vi "SPAN Stufen abfragen Gasteiler.vi"(5 "GD Info Cluster":T1, 6 "Sprachliste":string[][](array[string]), 7 "Boolsche Stufen Flags Cluster":T11, 8 "error in (no error)":errorcluster caption="Fehler (Eingang, kein Fehler)", 9 "Index":T14, 10 "Referenzen Cluster":T12, 11 "SpanInletClusterArray in":T2[](array[typedef]) {"zusätzliche Zeitdauer Erster Punkt" min=30 step=1 format="%#_5g"; "Zeitdauer Stufen" format="%#_5g"; "Max Fehler" format="%#_5g"; "Anzahl Stufen" format="%#_5g"; "Komponenten"."Komponente 5"."Komponente:" items=["NO (350,3000) LP 191C", "NO2 (150) LP 191C (1of2)", "NO2 (2000) LP 191C (2of2)", "N2O (300) LP 191C (1of2)", "NH3 (300) LP 191C (1of2)", "NH3 (900,3000) LP 191C (2of2)", "HNCO (400) 191C", "H2O% (30) LP 191C", "Formaldehyde (70,500) LP 191C", "CO2 low% (4) LP 191C (2of2)", "CO2% (20) LP 191C (1of2)", "CO (700) LP 191C (1of3)", "CO% (1) LP 191C (2of3)", "Propylene (1000) LP 191C", "Aromatic HC C7 (500) LP 191C", "Ethylene (1000) LP 191C", "CH4 (250) LP 191C (1of2)", "CH4 (5000) LP 191C (2of2)", "Ethane (1000) LP 191C", "Acetylene (1000) LP 191C", "HNO2 (20) 191C", "MeOH (1000) 191C", "CO% (10) LP 191C (3of3)", "Formic Acid (100) 191C", "SO2 (500) LP 191C", "Acetaldehyde (1000) LP 191C", "COS (100) LP 191C", "1,3 butadiene (100) LP 191C", "Oil as Octane (200) LP 191C", "N2O (1000) LP 191C (2of2)", "Propane (200) LP 191C", "NO2 autorange (2000)", "CO autorange (100000)", "CH4 autorange (5000)", "NH3 autorange (3000)", "Temp. Gascell", "Pressure Gascell", "sBeam@2500"]; "Komponenten"."Komponente 5"."Konzentration IST" format="%#.4f"; "Komponenten"."Komponente 5"."Genauigkeit" format="%#.1f"; "Komponenten"."Komponente 4"."Komponente:" items=["NO (350,3000) LP 191C", "NO2 (150) LP 191C (1of2)", "NO2 (2000) LP 191C (2of2)", "N2O (300) LP 191C (1of2)", "NH3 (300) LP 191C (1of2)", "NH3 (900,3000) LP 191C (2of2)", "HNCO (400) 191C", "H2O% (30) LP 191C", "Formaldehyde (70,500) LP 191C", "CO2 low% (4) LP 191C (2of2)", "CO2% (20) LP 191C (1of2)", "CO (700) LP 191C (1of3)", "CO% (1) LP 191C (2of3)", "Propylene (1000) LP 191C", "Aromatic HC C7 (500) LP 191C", "Ethylene (1000) LP 191C", "CH4 (250) LP 191C (1of2)", "CH4 (5000) LP 191C (2of2)", "Ethane (1000) LP 191C", "Acetylene (1000) LP 191C", "HNO2 (20) 191C", "MeOH (1000) 191C", "CO% (10) LP 191C (3of3)", "Formic Acid (100) 191C", "SO2 (500) LP 191C", "Acetaldehyde (1000) LP 191C", "COS (100) LP 191C", "1,3 butadiene (100) LP 191C", "Oil as Octane (200) LP 191C", "N2O (1000) LP 191C (2of2)", "Propane (200) LP 191C", "NO2 autorange (2000)", "CO autorange (100000)", "CH4 autorange (5000)", "NH3 autorange (3000)", "Temp. Gascell", "Pressure Gascell", "sBeam@2500"]; "Komponenten"."Komponente 4"."Konzentration IST" format="%#.4f"; "Komponenten"."Komponente 4"."Genauigkeit" format="%#.1f"; "Komponenten"."Komponente 3"."Komponente:" items=["NO (350,3000) LP 191C", "NO2 (150) LP 191C (1of2)", "NO2 (2000) LP 191C (2of2)", "N2O (300) LP 191C (1of2)", "NH3 (300) LP 191C (1of2)", "NH3 (900,3000) LP 191C (2of2)", "HNCO (400) 191C", "H2O% (30) LP 191C", "Formaldehyde (70,500) LP 191C", "CO2 low% (4) LP 191C (2of2)", "CO2% (20) LP 191C (1of2)", "CO (700) LP 191C (1of3)", "CO% (1) LP 191C (2of3)", "Propylene (1000) LP 191C", "Aromatic HC C7 (500) LP 191C", "Ethylene (1000) LP 191C", "CH4 (250) LP 191C (1of2)", "CH4 (5000) LP 191C (2of2)", "Ethane (1000) LP 191C", "Acetylene (1000) LP 191C", "HNO2 (20) 191C", "MeOH (1000) 191C", "CO% (10) LP 191C (3of3)", "Formic Acid (100) 191C", "SO2 (500) LP 191C", "Acetaldehyde (1000) LP 191C", "COS (100) LP 191C", "1,3 butadiene (100) LP 191C", "Oil as Octane (200) LP 191C", "N2O (1000) LP 191C (2of2)", "Propane (200) LP 191C", "NO2 autorange (2000)", "CO autorange (100000)", "CH4 autorange (5000)", "NH3 autorange (3000)", "Temp. Gascell", "Pressure Gascell", "sBeam@2500"]; "Komponenten"."Komponente 3"."Konzentration IST" format="%#.4f"; "Komponenten"."Komponente 3"."Genauigkeit" format="%#.1f"; "Komponenten"."Komponente 2"."Komponente:" items=["NO (350,3000) LP 191C", "NO2 (150) LP 191C (1of2)", "NO2 (2000) LP 191C (2of2)", "N2O (300) LP 191C (1of2)", "NH3 (300) LP 191C (1of2)", "NH3 (900,3000) LP 191C (2of2)", "HNCO (400) 191C", "H2O% (30) LP 191C", "Formaldehyde (70,500) LP 191C", "CO2 low% (4) LP 191C (2of2)", "CO2% (20) LP 191C (1of2)", "CO (700) LP 191C (1of3)", "CO% (1) LP 191C (2of3)", "Propylene (1000) LP 191C", "Aromatic HC C7 (500) LP 191C", "Ethylene (1000) LP 191C", "CH4 (250) LP 191C (1of2)", "CH4 (5000) LP 191C (2of2)", "Ethane (1000) LP 191C", "Acetylene (1000) LP 191C", "HNO2 (20) 191C", "MeOH (1000) 191C", "CO% (10) LP 191C (3of3)", "Formic Acid (100) 191C", "SO2 (500) LP 191C", "Acetaldehyde (1000) LP 191C", "COS (100) LP 191C", "1,3 butadiene (100) LP 191C", "Oil as Octane (200) LP 191C", "N2O (1000) LP 191C (2of2)", "Propane (200) LP 191C", "NO2 autorange (2000)", "CO autorange (100000)", "CH4 autorange (5000)", "NH3 autorange (3000)", "Temp. Gascell", "Pressure Gascell", "sBeam@2500"]; "Komponenten"."Komponente 2"."Konzentration IST" format="%#.4f"; "Komponenten"."Komponente 2"."Genauigkeit" format="%#.1f"; "Komponenten"."Komponente 1"."Komponente:" items=["NO (350,3000) LP 191C", "NO2 (150) LP 191C (1of2)", "NO2 (2000) LP 191C (2of2)", "N2O (300) LP 191C (1of2)", "NH3 (300) LP 191C (1of2)", "NH3 (900,3000) LP 191C (2of2)", "HNCO (400) 191C", "H2O% (30) LP 191C", "Formaldehyde (70,500) LP 191C", "CO2 low% (4) LP 191C (2of2)", "CO2% (20) LP 191C (1of2)", "CO (700) LP 191C (1of3)", "CO% (1) LP 191C (2of3)", "Propylene (1000) LP 191C", "Aromatic HC C7 (500) LP 191C", "Ethylene (1000) LP 191C", "CH4 (250) LP 191C (1of2)", "CH4 (5000) LP 191C (2of2)", "Ethane (1000) LP 191C", "Acetylene (1000) LP 191C", "HNO2 (20) 191C", "MeOH (1000) 191C", "CO% (10) LP 191C (3of3)", "Formic Acid (100) 191C", "SO2 (500) LP 191C", "Acetaldehyde (1000) LP 191C", "COS (100) LP 191C", "1,3 butadiene (100) LP 191C", "Oil as Octane (200) LP 191C", "N2O (1000) LP 191C (2of2)", "Propane (200) LP 191C", "NO2 autorange (2000)", "CO autorange (100000)", "CH4 autorange (5000)", "NH3 autorange (3000)", "Temp. Gascell", "Pressure Gascell", "sBeam@2500"]; "Komponenten"."Komponente 1"."Konzentration IST" format="%#.4f"; "Komponenten"."Komponente 1"."Genauigkeit" format="%#.1f"; "Ablaufdatum" format="%<%d.%m.%Y>T"; "Gasflasche" items=["----"=10000, "IAG NH3 3000"=0, "IAG NH3 200"=1, "IAG NH3 2000"=2, "IAG MG"=3, "IAG O2"=4]}) -> (0 "error out":errorcluster caption="Fehler (Ausgang)", 1 "Component Index out":i32, 2 "SPAN Index out":i32, 3 "SpanInletClusterArray out":T2[](array[typedef]) {"zusätzliche Zeitdauer Erster Punkt" min=30 step=1 format="%#_5g"; "Zeitdauer Stufen" format="%#_5g"; "Max Fehler" format="%#_5g"; "Anzahl Stufen" format="%#_5g"; "Komponenten"."Komponente 5"."Komponente:" items=["NO (350,3000) LP 191C", "NO2 (150) LP 191C (1of2)", "NO2 (2000) LP 191C (2of2)", "N2O (300) LP 191C (1of2)", "NH3 (300) LP 191C (1of2)", "NH3 (900,3000) LP 191C (2of2)", "HNCO (400) 191C", "H2O% (30) LP 191C", "Formaldehyde (70,500) LP 191C", "CO2 low% (4) LP 191C (2of2)", "CO2% (20) LP 191C (1of2)", "CO (700) LP 191C (1of3)", "CO% (1) LP 191C (2of3)", "Propylene (1000) LP 191C", "Aromatic HC C7 (500) LP 191C", "Ethylene (1000) LP 191C", "CH4 (250) LP 191C (1of2)", "CH4 (5000) LP 191C (2of2)", "Ethane (1000) LP 191C", "Acetylene (1000) LP 191C", "HNO2 (20) 191C", "MeOH (1000) 191C", "CO% (10) LP 191C (3of3)", "Formic Acid (100) 191C", "SO2 (500) LP 191C", "Acetaldehyde (1000) LP 191C", "COS (100) LP 191C", "1,3 butadiene (100) LP 191C", "Oil as Octane (200) LP 191C", "N2O (1000) LP 191C (2of2)", "Propane (200) LP 191C", "NO2 autorange (2000)", "CO autorange (100000)", "CH4 autorange (5000)", "NH3 autorange (3000)", "Temp. Gascell", "Pressure Gascell", "sBeam@2500"]; "Komponenten"."Komponente 5"."Konzentration IST" format="%#.4f"; "Komponenten"."Komponente 5"."Genauigkeit" format="%#.1f"; "Komponenten"."Komponente 4"."Komponente:" items=["NO (350,3000) LP 191C", "NO2 (150) LP 191C (1of2)", "NO2 (2000) LP 191C (2of2)", "N2O (300) LP 191C (1of2)", "NH3 (300) LP 191C (1of2)", "NH3 (900,3000) LP 191C (2of2)", "HNCO (400) 191C", "H2O% (30) LP 191C", "Formaldehyde (70,500) LP 191C", "CO2 low% (4) LP 191C (2of2)", "CO2% (20) LP 191C (1of2)", "CO (700) LP 191C (1of3)", "CO% (1) LP 191C (2of3)", "Propylene (1000) LP 191C", "Aromatic HC C7 (500) LP 191C", "Ethylene (1000) LP 191C", "CH4 (250) LP 191C (1of2)", "CH4 (5000) LP 191C (2of2)", "Ethane (1000) LP 191C", "Acetylene (1000) LP 191C", "HNO2 (20) 191C", "MeOH (1000) 191C", "CO% (10) LP 191C (3of3)", "Formic Acid (100) 191C", "SO2 (500) LP 191C", "Acetaldehyde (1000) LP 191C", "COS (100) LP 191C", "1,3 butadiene (100) LP 191C", "Oil as Octane (200) LP 191C", "N2O (1000) LP 191C (2of2)", "Propane (200) LP 191C", "NO2 autorange (2000)", "CO autorange (100000)", "CH4 autorange (5000)", "NH3 autorange (3000)", "Temp. Gascell", "Pressure Gascell", "sBeam@2500"]; "Komponenten"."Komponente 4"."Konzentration IST" format="%#.4f"; "Komponenten"."Komponente 4"."Genauigkeit" format="%#.1f"; "Komponenten"."Komponente 3"."Komponente:" items=["NO (350,3000) LP 191C", "NO2 (150) LP 191C (1of2)", "NO2 (2000) LP 191C (2of2)", "N2O (300) LP 191C (1of2)", "NH3 (300) LP 191C (1of2)", "NH3 (900,3000) LP 191C (2of2)", "HNCO (400) 191C", "H2O% (30) LP 191C", "Formaldehyde (70,500) LP 191C", "CO2 low% (4) LP 191C (2of2)", "CO2% (20) LP 191C (1of2)", "CO (700) LP 191C (1of3)", "CO% (1) LP 191C (2of3)", "Propylene (1000) LP 191C", "Aromatic HC C7 (500) LP 191C", "Ethylene (1000) LP 191C", "CH4 (250) LP 191C (1of2)", "CH4 (5000) LP 191C (2of2)", "Ethane (1000) LP 191C", "Acetylene (1000) LP 191C", "HNO2 (20) 191C", "MeOH (1000) 191C", "CO% (10) LP 191C (3of3)", "Formic Acid (100) 191C", "SO2 (500) LP 191C", "Acetaldehyde (1000) LP 191C", "COS (100) LP 191C", "1,3 butadiene (100) LP 191C", "Oil as Octane (200) LP 191C", "N2O (1000) LP 191C (2of2)", "Propane (200) LP 191C", "NO2 autorange (2000)", "CO autorange (100000)", "CH4 autorange (5000)", "NH3 autorange (3000)", "Temp. Gascell", "Pressure Gascell", "sBeam@2500"]; "Komponenten"."Komponente 3"."Konzentration IST" format="%#.4f"; "Komponenten"."Komponente 3"."Genauigkeit" format="%#.1f"; "Komponenten"."Komponente 2"."Komponente:" items=["NO (350,3000) LP 191C", "NO2 (150) LP 191C (1of2)", "NO2 (2000) LP 191C (2of2)", "N2O (300) LP 191C (1of2)", "NH3 (300) LP 191C (1of2)", "NH3 (900,3000) LP 191C (2of2)", "HNCO (400) 191C", "H2O% (30) LP 191C", "Formaldehyde (70,500) LP 191C", "CO2 low% (4) LP 191C (2of2)", "CO2% (20) LP 191C (1of2)", "CO (700) LP 191C (1of3)", "CO% (1) LP 191C (2of3)", "Propylene (1000) LP 191C", "Aromatic HC C7 (500) LP 191C", "Ethylene (1000) LP 191C", "CH4 (250) LP 191C (1of2)", "CH4 (5000) LP 191C (2of2)", "Ethane (1000) LP 191C", "Acetylene (1000) LP 191C", "HNO2 (20) 191C", "MeOH (1000) 191C", "CO% (10) LP 191C (3of3)", "Formic Acid (100) 191C", "SO2 (500) LP 191C", "Acetaldehyde (1000) LP 191C", "COS (100) LP 191C", "1,3 butadiene (100) LP 191C", "Oil as Octane (200) LP 191C", "N2O (1000) LP 191C (2of2)", "Propane (200) LP 191C", "NO2 autorange (2000)", "CO autorange (100000)", "CH4 autorange (5000)", "NH3 autorange (3000)", "Temp. Gascell", "Pressure Gascell", "sBeam@2500"]; "Komponenten"."Komponente 2"."Konzentration IST" format="%#.4f"; "Komponenten"."Komponente 2"."Genauigkeit" format="%#.1f"; "Komponenten"."Komponente 1"."Komponente:" items=["NO (350,3000) LP 191C", "NO2 (150) LP 191C (1of2)", "NO2 (2000) LP 191C (2of2)", "N2O (300) LP 191C (1of2)", "NH3 (300) LP 191C (1of2)", "NH3 (900,3000) LP 191C (2of2)", "HNCO (400) 191C", "H2O% (30) LP 191C", "Formaldehyde (70,500) LP 191C", "CO2 low% (4) LP 191C (2of2)", "CO2% (20) LP 191C (1of2)", "CO (700) LP 191C (1of3)", "CO% (1) LP 191C (2of3)", "Propylene (1000) LP 191C", "Aromatic HC C7 (500) LP 191C", "Ethylene (1000) LP 191C", "CH4 (250) LP 191C (1of2)", "CH4 (5000) LP 191C (2of2)", "Ethane (1000) LP 191C", "Acetylene (1000) LP 191C", "HNO2 (20) 191C", "MeOH (1000) 191C", "CO% (10) LP 191C (3of3)", "Formic Acid (100) 191C", "SO2 (500) LP 191C", "Acetaldehyde (1000) LP 191C", "COS (100) LP 191C", "1,3 butadiene (100) LP 191C", "Oil as Octane (200) LP 191C", "N2O (1000) LP 191C (2of2)", "Propane (200) LP 191C", "NO2 autorange (2000)", "CO autorange (100000)", "CH4 autorange (5000)", "NH3 autorange (3000)", "Temp. Gascell", "Pressure Gascell", "sBeam@2500"]; "Komponenten"."Komponente 1"."Konzentration IST" format="%#.4f"; "Komponenten"."Komponente 1"."Genauigkeit" format="%#.1f"; "Ablaufdatum" format="%<%d.%m.%Y>T"; "Gasflasche" items=["----"=10000, "IAG NH3 3000"=0, "IAG NH3 200"=1, "IAG NH3 2000"=2, "IAG MG"=3, "IAG O2"=4]}, 4 "Status out":string)   [LabVIEW 2020, in "Linearisierung v2.lvlib" / "SpanEinstellungen.lvlib"]
uses:
  SpanEinstellungen.lvlib
  Visualisierungs Elemente/Checkbox(boolsch).ctl
  GD Abfrage Referenzen.ctl
  Boolsche Stufen Flags.ctl
  SpanInletCluster.ctl
  Seiten/System Einstellungen V2/Konfig Gasflasche.ctl
  Seiten/System Einstellungen V2/Analysatoren.ctl
  Seiten/System Einstellungen V2/Gasflasche Auswahl.ctl
  Komponentencluster mit Formel.ctl
  Komponentenauswahl mit Formel.ctl
  Visualisierungs Elemente/String - Eingabefeld.ctl
  Einheit.ctl
  Seiten/System Einstellungen V2/Traegergas.ctl
  GasteilerType.ctl
  Gasteiler/Aktionen FGV Gasteiler Daten.ctl
  Linearisierung v2.lvlib
  Gasteiler/Gasteiler.lvlib
  Sprachverwaltung/Sprachverwaltung.lvlib
  Seiten/System Einstellungen V2/System Einstellungen V2.lvlib
panel:
  # "sec"
  # "%"
  # "sec"
  # "Komponente"
  # "Formel"
  # "Konzentration"
  # "Einheit"
  # "Genauigkeit [%]"
  # "sec"
  # "%"
  # "sec"
  # "Komponente"
  # "Formel"
  # "Konzentration"
  # "Einheit"
  # "Genauigkeit [%]"
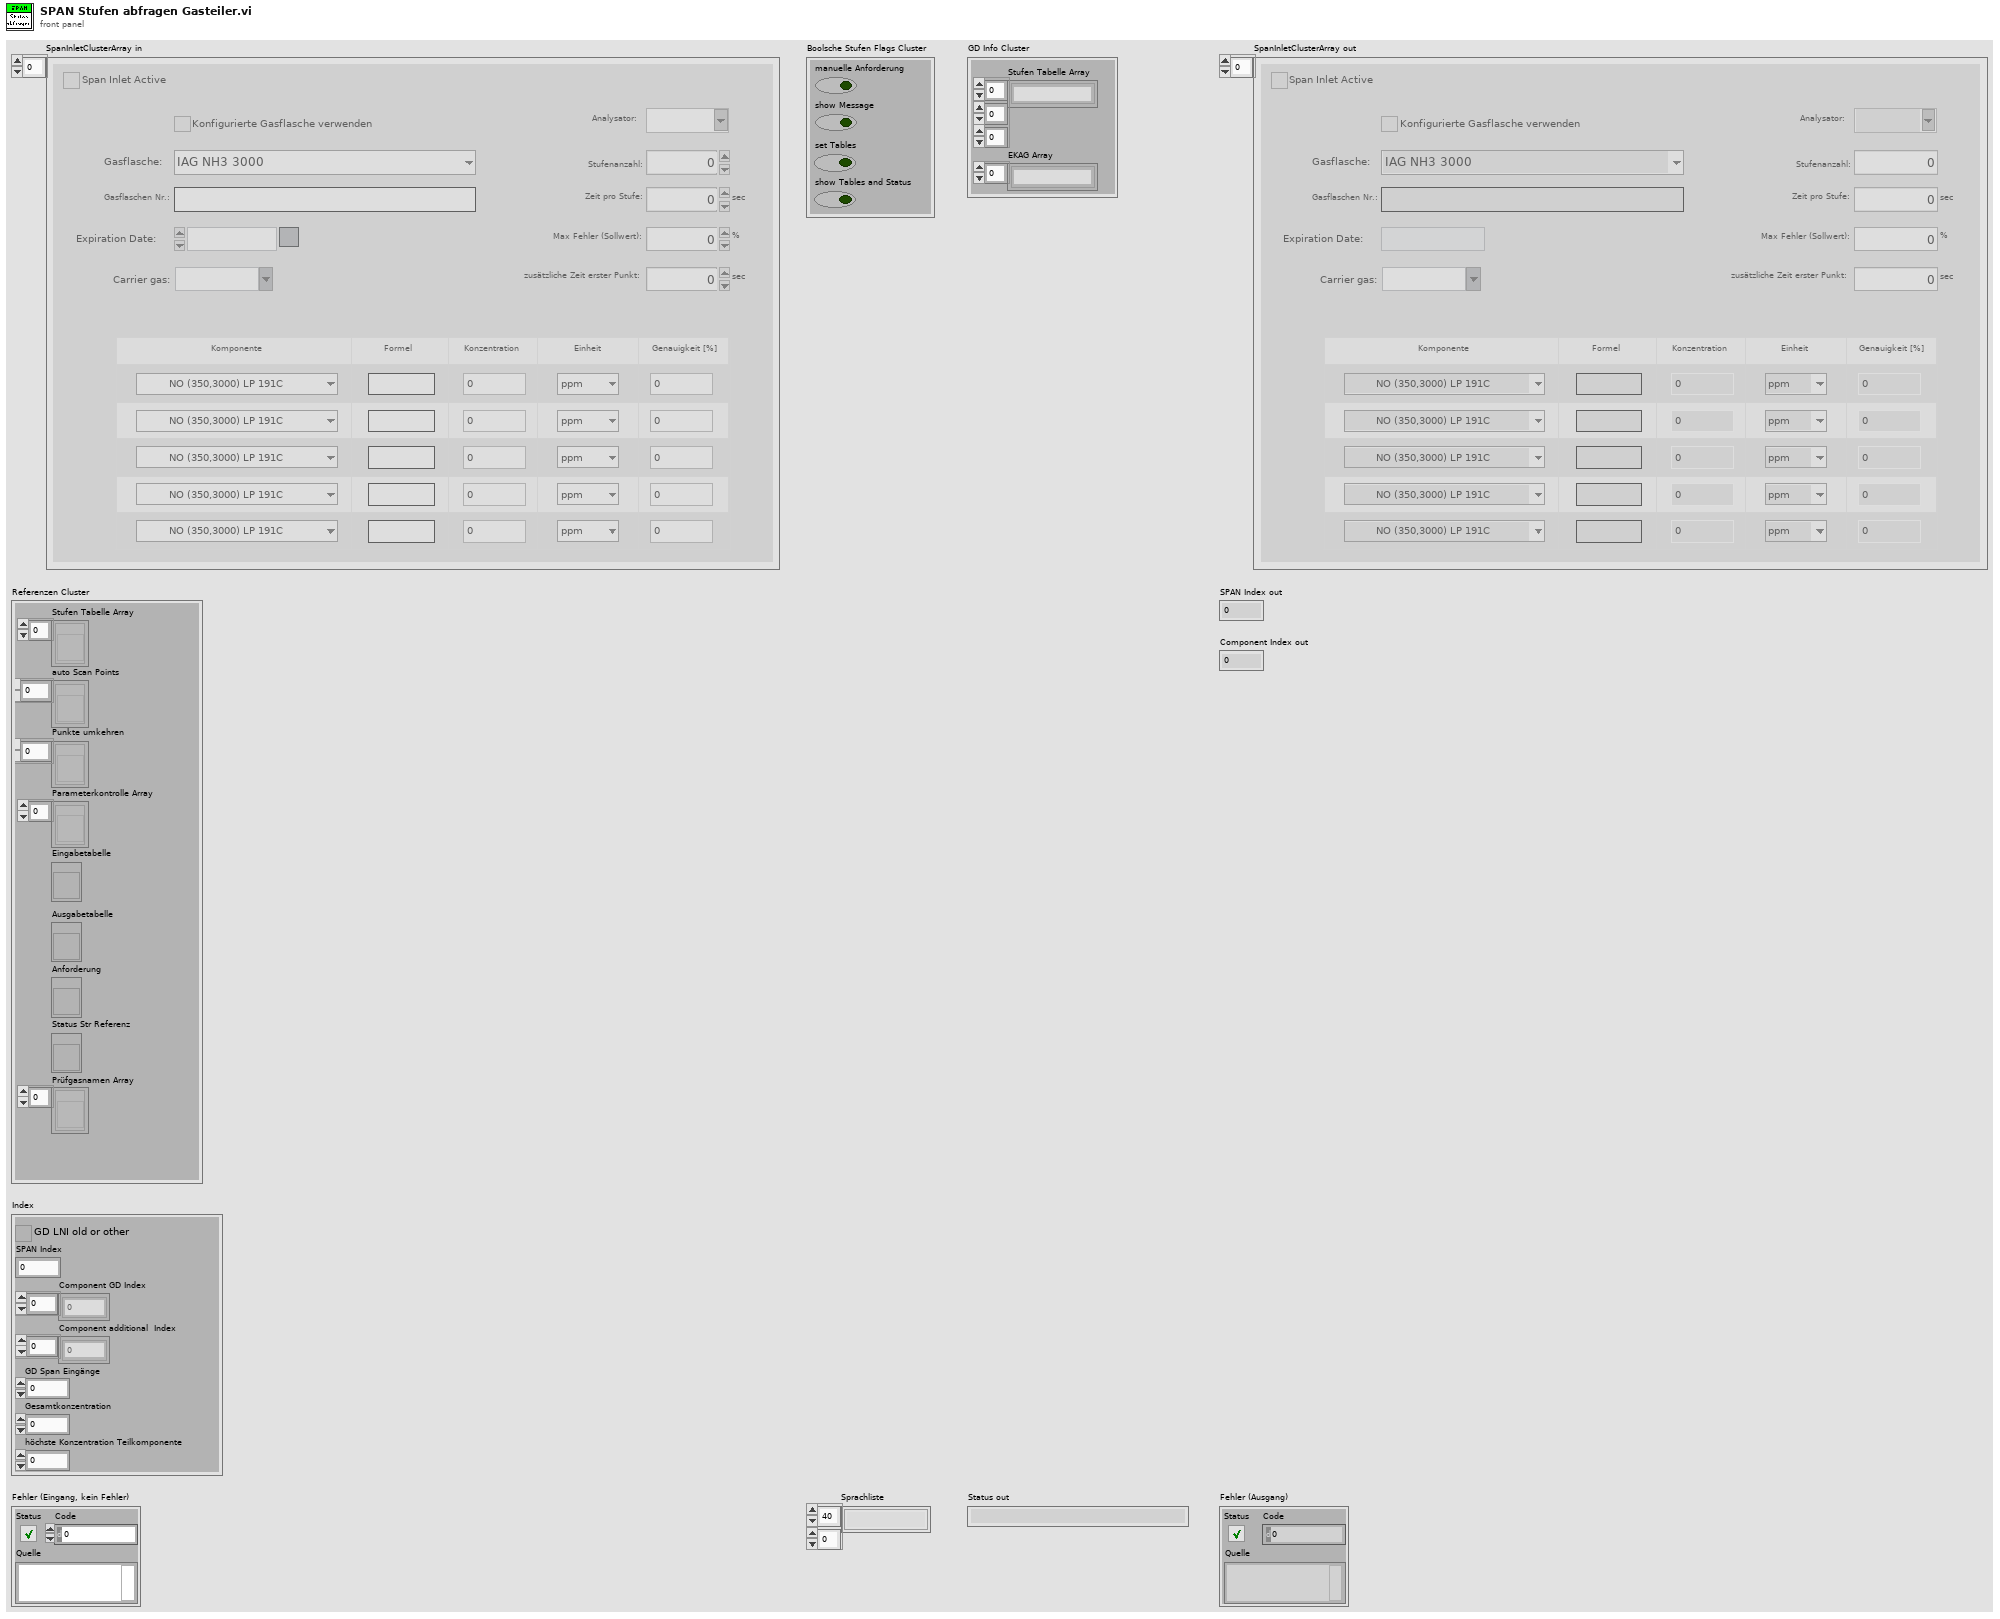
[diagram p1: front panel]
types:
  T1 = cluster{"Stufen Tabelle Array":string[][][], "EKAG Array":string[]}
  T2 = typedef "Linearisierung v2.lvlib/SpanEinstellungen.lvlib/SpanInletCluster.ctl" = cluster{"Span Inlet Active":T3, "Analysator":T4, "Konfig Gasflasche":T3, "Gasflasche":T5, "Gasflaschen Nr.:":string, "Ablaufdatum":timestamp, "Komponenten":T6, "Zeitdauer Stufen":sgl, "Max Fehler":sgl, "Anzahl Stufen":sgl, "Trägergas":T10, "zusätzliche Zeitdauer Erster Punkt":sgl}
  T3 = typedef "System Einstellungen V2.lvlib/Konfig Gasflasche.ctl" = bool
  T4 = typedef "System Einstellungen V2.lvlib/Analysatoren.ctl" = string
  T5 = typedef "System Einstellungen V2.lvlib/Gasflasche Auswahl.ctl" = u16
  T6 = typedef "Linearisierung v2.lvlib/SpanEinstellungen.lvlib/Komponentencluster mit Formel.ctl" = cluster{"Komponente 1":T7, "Komponente 2":T7, "Komponente 3":T7, "Komponente 4":T7, "Komponente 5":T7}
  T7 = typedef "Linearisierung v2.lvlib/SpanEinstellungen.lvlib/Komponentenauswahl mit Formel.ctl" = cluster{"Komponente:":u16, "Summenformel":T8, "Konzentration IST":dbl, "Einheit":T9, "Genauigkeit":dbl}
  T8 = typedef "String - Eingabefeld.ctl" = string
  T9 = typedef "Linearisierung v2.lvlib/SpanEinstellungen.lvlib/Einheit.ctl" = enum16{"ppm", "%"}
  T10 = typedef "System Einstellungen V2.lvlib/Traegergas.ctl" = string
  T11 = typedef "Linearisierung v2.lvlib/SpanEinstellungen.lvlib/Boolsche Stufen Flags.ctl" = cluster{"manuelle Anforderung":bool, "show Message":bool, "set Tables":bool, "show Tables and Status":bool}
  T12 = typedef "Linearisierung v2.lvlib/SpanEinstellungen.lvlib/GD Abfrage Referenzen.ctl" = cluster{"Stufen Tabelle Array":refnum<vi>[], "auto Scan Points":refnum<vi>[], "Punkte umkehren":refnum<vi>[], "Parameterkontrolle Array":refnum<vi>[], "Eingabetabelle":refnum<vi>, "Ausgabetabelle":refnum<vi>, "Anforderung":refnum<vi>, "Status Str Referenz":refnum<vi>, "Prüfgasnamen Array":refnum<vi>[]}
  T13 = typedef "Checkbox(boolsch).ctl" = bool
  T14 = cluster{"GD LNI old or other":T13, "SPAN Index":i32, "Component GD Index":i32[], "Component additional  Index":i32[], "GD Span Eingänge":u16, "Gesamtkonzentration":dbl, "höchste Konzentration Teilkomponente":dbl}
  T15 = typedef "Linearisierung v2.lvlib/Gasteiler.lvlib/Aktionen FGV Gasteiler Daten.ctl" = enum16{"lesen", "Gasteiler Daten", "Seriellen Param.", "MB-Endwert", "laden", "speichern", "Anforderung", "TCP", "Aufzeichnung Start"}
  T16 = typedef "Linearisierung v2.lvlib/GasteilerType.ctl" = u16
  T17 = typedef "Linearisierung v2.lvlib/Gasteiler.lvlib/Gasteiler Daten.ctl" = cluster{"Gasteiler":T8, "Gasteiler Stufen":T18, "Gasteiler Type":T16, "Konfig Gasteiler":T19, "Gasteiler Span Eingänge":u16}
  T18 = typedef "Linearisierung v2.lvlib/Gasteiler.lvlib/Gasteiler Stufen.ctl" = u16
  T19 = typedef "System Einstellungen V2.lvlib/Gasteiler Auswahl.ctl" = u16
  T20 = typedef "Button.ctl" = bool
  T21 = cluster{"Komponente:":u16, "Konzentration IST":dbl}[]
  T22 = typedef "Linearisierung v2.lvlib/Gasteiler.lvlib/Prüfgas in.ctl" = u16
  T23 = cluster{"GD LNI old or other":T13, "Anzahl Stufen":sgl, "Verdünnungsgas":T22, "Component GD Index":i32[], "Component additional  Index":i32[], "DIL Input":i32}
  T24 = cluster{"manuelle Anforderung":bool, "show Tables and Status":bool}
  T25 = cluster{"Stufen Tabellen out":string[][][], "EGAK":T10[], "AGAK":string[]}
  T26 = cluster{"SPAN Index":i32, "Component Index out":i32}
  T27 = cluster{i32, cluster{"SPAN Index":i32, "Component Index out":i32}}
  T28 = cluster{bool, bool, "Gesamtkonzentration":dbl, "höchste Konzentration Teilkomponente":dbl}
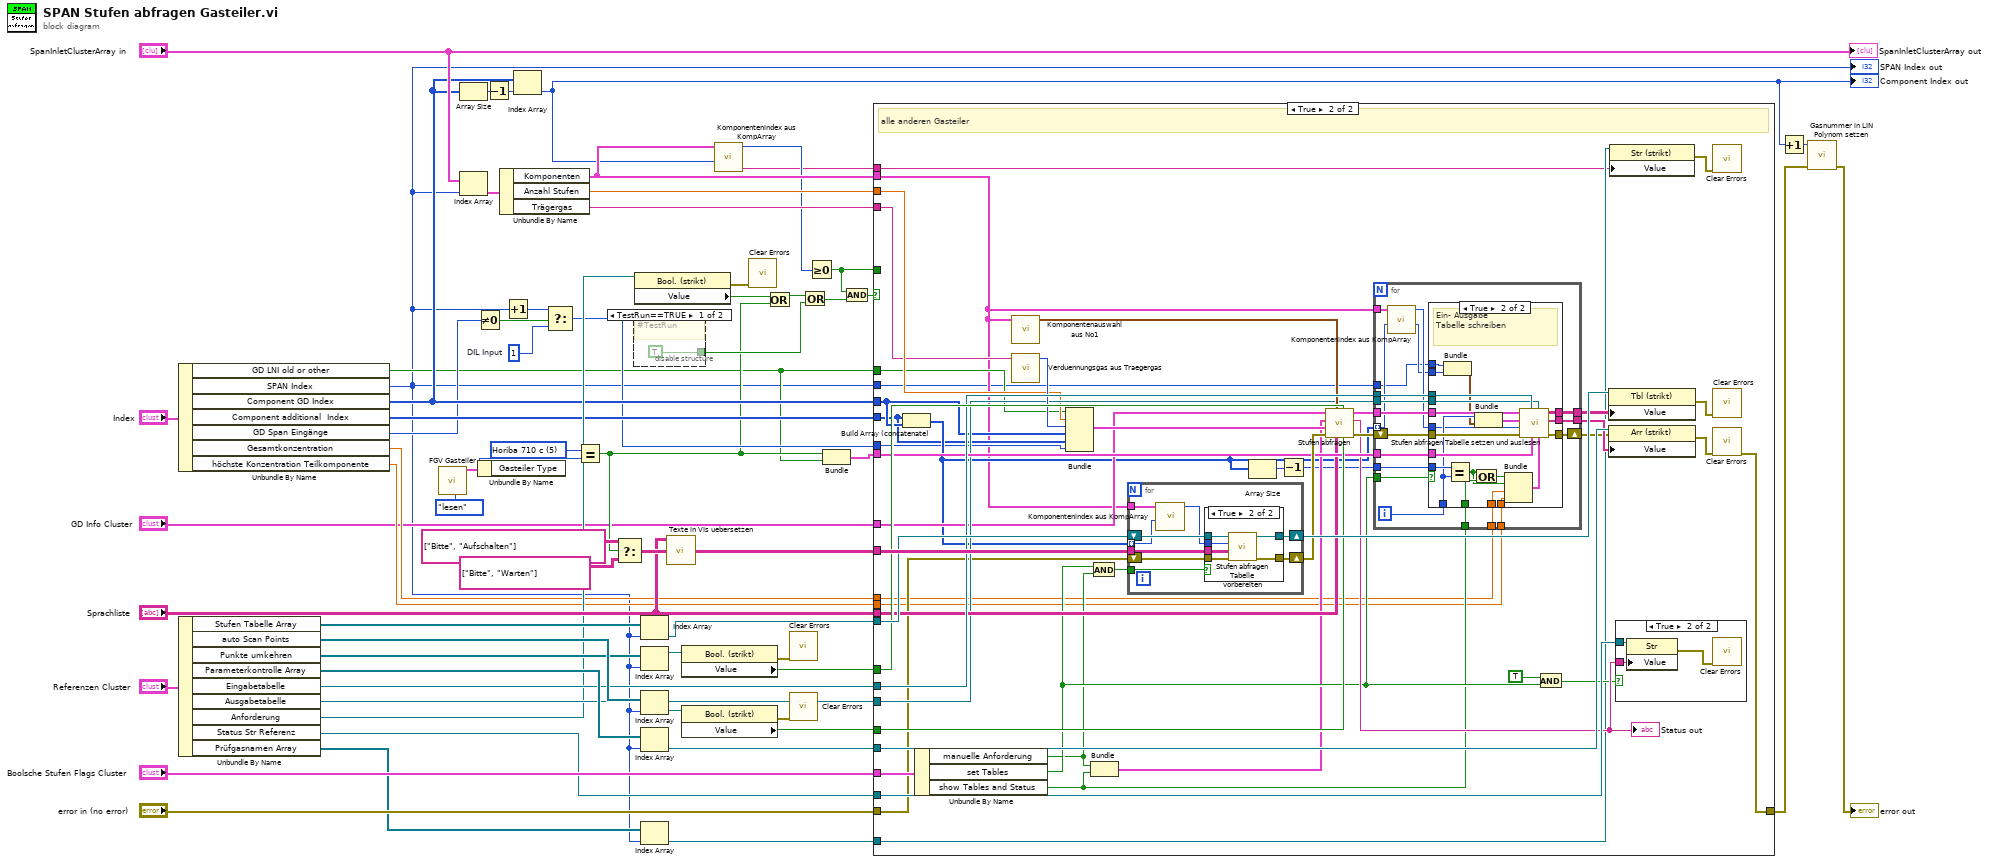
[diagram p0: block diagram]
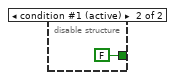
[diagram p2: hidden frame]
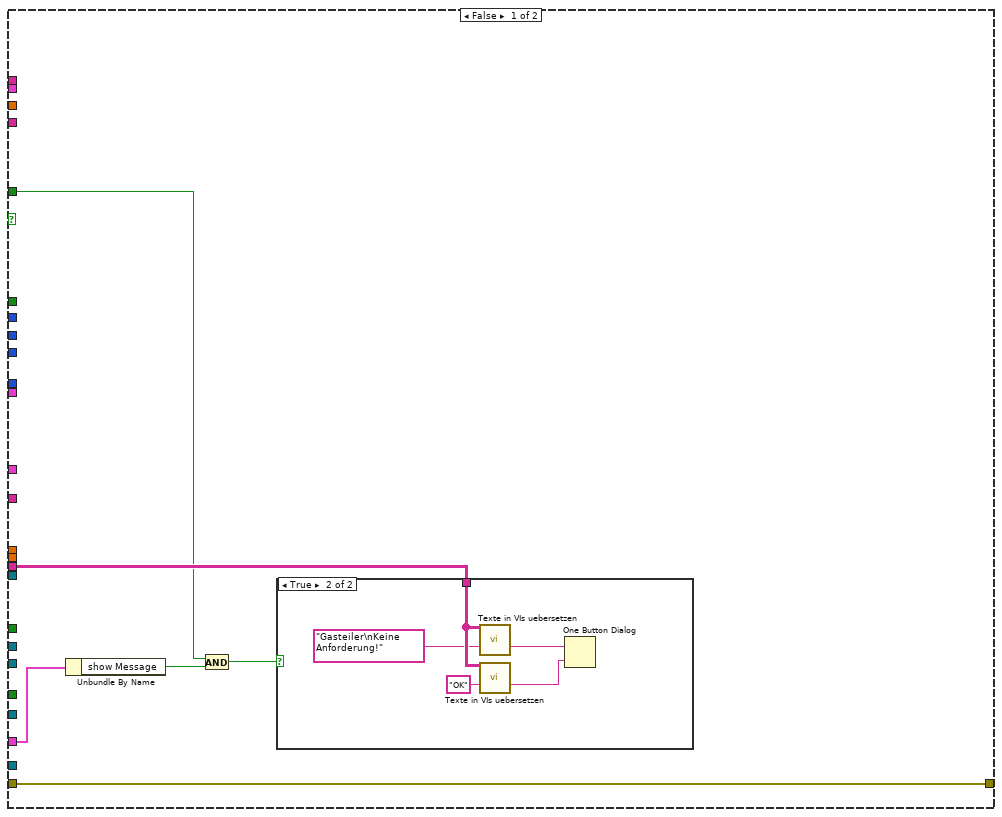
[diagram p3: hidden frame]
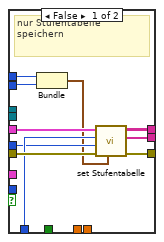
[diagram p5: hidden frame]
diagram:
  w17 = 1  # DIL Input
  w61 = T16 5 items=["LCD-Touch-Display", "Analog-Display", "AVL GDU", "Horiba GDC", "HovaCal", "Horiba 710 c"] ("x")
  n1 = Unbundle By Name("Index") -> ("GD LNI old or other"=w5:T13, "SPAN Index"=w1:i32, "Component GD Index"=w24:i32[], "Component additional  Index"=w25:i32[], "GD Span Eingänge"=w19:u16, "Gesamtkonzentration"=w12:dbl, "höchste Konzentration Teilkomponente"=w11:dbl)
  "SPAN Index out" <- w1
  n2 = Unbundle By Name("Referenzen Cluster") -> ("Stufen Tabelle Array"=w55:refnum<vi>[], "auto Scan Points"=w54:refnum<vi>[], "Punkte umkehren"=w53:refnum<vi>[], "Parameterkontrolle Array"=w52:refnum<vi>[], "Eingabetabelle"=w51:refnum<vi>, "Ausgabetabelle"=w35:refnum<vi>, "Anforderung"=w32:refnum<vi>, "Status Str Referenz"=w33:refnum<vi>, "Prüfgasnamen Array"=w14:refnum<vi>[])
  n3 = call "FGV Gasteiler.vi"("Aktionen"=Aktionen_FGV_Gasteiler_Daten."lesen") -> ("Gasteiler Daten"=w62:T17)  [unwired: 11 in, 7 out]
  n4 = Array Size(array=w24) -> (size(s)=w23:i32)
  n5 = Index Array(array="SpanInletClusterArray in", index=w1) -> (element=w30:T2)
  n6 = Not Equal To 0?(x=w19) -> (x != 0?=w18:bool)
  n7 = Unbundle By Name(w62) -> ("Gasteiler Type"=w64:T16)
  n8 = Decrement(x=w23) -> (x-1=w22:i32)
  n9 = Unbundle By Name(w30) -> ("Komponenten"=w21:T6, "Anzahl Stufen"=w29:sgl, "Trägergas"=w28:T10)
  n10 = Increment(x=w1) -> (x+1=w15:i32)
  n11 = Index Array(array=w24, index=w22) -> (element=w10:i32)
  "Component Index out" <- w10
  n12 = Select(t=w15, s=w18, f=w17) -> (s? t:f=w16:i32)
  n13 = Equal?(x=w61, y=w64) -> (x = y?=w6:bool)
  n14 = Select(t=string[][] [["Bitte", "Aufschalten"]] ("Stufen Tabelle"), s=w6, f=string[][] [["Bitte", "Warten"]] ("Stufen Tabelle")) -> (s? t:f=w47:string[][])
  n15 = disable-structure shown="TestRun==TRUE" {
    disable-tunnel: [TRUE FALSE] -> w36
    frame condition #0 {
      # "#TestRun"
    }
    frame condition #1 (active) {
    }
  }
  n16 = property class="Bool. (strikt)"(reference=w32) -> (error out=w41:errorcluster, "Value"=w42:T20)  [unwired: 1 in, 1 out]
  n17 = Index Array(array=w55, index=w1) -> (element=w39:refnum<vi>)
  n18 = Index Array(array=w53, index=w1) -> (element=w60:refnum<vi>)
  n19 = Index Array(array=w54, index=w1) -> (element=w49:refnum<vi>)
  n20 = Index Array(array=w52, index=w1) -> (element=w65:refnum<vi>)
  n21 = Index Array(array=w14, index=w1) -> (element=w13:refnum<vi>)
  n22 = call "Texte in VIs uebersetzen.vi"("Sprachliste"="Sprachliste", "2D String-Array zum Übersetzen"=w47) -> ("2D String-Array zum Übersetzen"=w45:string[][])  [unwired: 9 in, 4 out]
  n23 = property class="Bool. (strikt)"(reference=w60) -> (error out=w58:errorcluster, "Value"=w59:bool)  [unwired: 1 in, 1 out]
  n24 = property class="Bool. (strikt)"(reference=w49) -> (error out=w50:errorcluster, "Value"=w48:bool)  [unwired: 1 in, 1 out]
  n25 = call "Komponentenindex aus KompArray.vi"("Component Index in"=w10, "Komponenten"=w21) -> ("Summenformel"=w2:T8, "Komponenten Index"=w20:u16)  [unwired: 7 in, 1 out]
  n26 = call <vilib>:"Clear Errors.vi"("error in (no error)"=w41) -> ()  [unwired: 5 in, 2 out]
  n27 = Or(x=w42, y=w6) -> (x .or. y?=w40:T20)
  n28 = call <vilib>:"Clear Errors.vi"("error in (no error)"=w58) -> ()  [unwired: 5 in, 2 out]
  n29 = call <vilib>:"Clear Errors.vi"("error in (no error)"=w50) -> ()  [unwired: 5 in, 2 out]
  n30 = Or(x=w40, y=w36) -> (x .or. y?=w37:T20)
  n31 = Greater Or Equal To 0?(x=w20) -> (x >= 0?=w26:bool)
  n32 = Bundle(w6, "GD LNI old or other"=w5) -> (w4:cluster{bool, "GD LNI old or other":T13})  [unwired: 1 in]
  n33 = And(x=w26, y=w37) -> (x .and. y?=w27:T20)
  n34 = case shown="True" w27 {
    tunnel: w65 -> [_ w127]
    tunnel: w51 -> [_ w118]
    tunnel: w59 -> [_ w120]
    tunnel: w24 -> [_ w92]
    tunnel: w48 -> [_ w121]
    tunnel: w45 -> [_ w124]
    tunnel: w4 -> [_ w117]
    tunnel: "Sprachliste" -> [w73 w108]
    tunnel: w39 -> [_ w123]
    tunnel: "Boolsche Stufen Flags Cluster" -> [w70 w104]
    tunnel: "error in (no error)" -> [w72 w99]
    tunnel: [w72 w112] -> w9
    tunnel: w33 -> [_ w107]
    tunnel: w35 -> [_ w105]
    tunnel: w21 -> [_ w83]
    tunnel: w29 -> [_ w98]
    tunnel: w28 -> [_ w97]
    tunnel: w26 -> [w68 _]
    tunnel: "GD Info Cluster" -> [_ w93]
    tunnel: w5 -> [_ w94]
    tunnel: w25 -> [_ w87]
    tunnel: w16 -> [_ w86]
    tunnel: w13 -> [_ w84]
    tunnel: w2 -> [_ w82]
    tunnel: w12 -> [_ w81]
    tunnel: w11 -> [_ w80]
    tunnel: w1 -> [_ w79]
    frame False {
      n35 = Unbundle By Name(w70) -> ("show Message"=w71:bool)
      n36 = And(x=w68, y=w71) -> (x .and. y?=w69:bool)
      n37 = case shown="True" w69 {
        tunnel: w73 -> [_ w78]
        frame False {
        }
        frame True {
          n38 = call "Texte in VIs uebersetzen.vi"("Sprachliste"=w78, "String zum Übersetzen"="Gasteiler\nKeine Anforderung!" ("Nachricht")) -> ("String zum Übersetzen"=w76:string)  [unwired: 9 in, 4 out]
          n39 = call "Texte in VIs uebersetzen.vi"("Sprachliste"=w78, "String zum Übersetzen"="OK") -> ("String zum Übersetzen"=w75:string)  [unwired: 9 in, 4 out]
          n40 = One Button Dialog(message=w76, button name ("OK")=w75) -> ()  [unwired: 1 out]
        }
      }
    }
    frame True {
      # "alle anderen Gasteiler"
      n41 = Build Array (concatenate)(w87, w92) -> (w90:i32[])
      n42 = Unbundle By Name(w104) -> ("manuelle Anforderung"=w95:bool, "set Tables"=w103:bool, "show Tables and Status"=w100:bool)
      n43 = call "Komponentenauswahl aus No1.vi"("Komponente 1"=w83) -> ("Komponentenauswahl"=w111:T21)  [unwired: 8 in, 2 out]
      n44 = call "Verduennungsgas aus Traegergas.vi"("Trägergas"=w97) -> ("Verdünnungsgas"=w110:T22)  [unwired: 10 in]
      n45 = Bundle("GD LNI old or other"=w94, "Anzahl Stufen"=w98, "Verdünnungsgas"=w110, "Component GD Index"=w92, "Component additional  Index"=w87, "DIL Input"=w86) -> (w109:T23)  [unwired: 1 in]
      n46 = And(x=w103, y=w95) -> (x .and. y?=w96:bool)
      n47 = Bundle("manuelle Anforderung"=w95, "show Tables and Status"=w100) -> (w102:T24)  [unwired: 1 in]
      n48 = for {
        tunnel: w124 -> [w185]
        tunnel: w90 -> [w179] mode=indexing
        tunnel: w96 -> [w181]
        shift-right: [w186] -> w128
        shift-left: w123 -> [w184]
        shift-right: [w183] -> w122
        shift-left: w99 -> [w182]
        tunnel: w83 -> [w180]
        n49 = call "Komponentenindex aus KompArray.vi"("Component Index in"=w179, "Komponenten"=w180) -> ("Komponenten Index"=w178:u16)  [unwired: 7 in, 2 out]
        n50 = case shown="True" w181 {
          tunnel: w178 -> [_ w194]
          tunnel: [w188 w193] -> w186
          tunnel: w185 -> [_ w192]
          tunnel: w184 -> [w188 w191]
          tunnel: [w187 w190] -> w183
          tunnel: w182 -> [w187 w189]
          frame False {
          }
          frame True {
            n51 = call "Stufen abfragen Tabelle vorbereiten.vi"("Fehler (Eingang)"=w189, "2D String-Array zum Übersetzen"=w192, "Komponente in"=w194, "Tabelle (Eingang)"=w191) -> ("Fehler (Ausgang)"=w190:errorcluster, "Tabelle (Ausgang)"=w193:refnum<vi>)  [unwired: 5 in, 1 out]
          }
        }
      }
      n52 = Array Size(array=w90) -> (size(s)=w89:i32)
      n53 = Decrement(x=w89) -> (x-1=w88:i32)
      n54 = call "Stufen abfragen.vi"("auto Scan Points"=w121, "Punkte umkehren"=w120, "Sprachliste"=w108, "Komponentenauswahl"=w111, "error in (no error)"=w122, "Index Cluster"=w109, "Bollche Flags Cluster"=w102, "GD Info Cluster"=w93) -> ("error out"=w119:errorcluster, "Status out"=w106:string, "GD out"=w116:T25)  [unwired: 1 out]
      "Status out" <- w106
      n55 = for {
        tunnel: w118 -> [w146]
        tunnel: w117 -> [w145]
        tunnel: w116 -> [w144]
        tunnel: w90 -> [w134] mode=indexing
        tunnel: [w143] -> w115
        tunnel: [w142] -> w114
        tunnel: w105 -> [w140]
        tunnel: w103 -> [w139]
        tunnel: w100 -> [w138]
        shift-right: [w141] -> w113
        shift-left: w119 -> [w147]
        tunnel: w88 -> [w136]
        tunnel: w83 -> [w135]
        tunnel: w81 -> [w132]
        tunnel: w80 -> [w131]
        tunnel: w79 -> [w129]
        i -> [w137]
        n56 = call "Komponentenindex aus KompArray.vi"("Component Index in"=w134, "Komponenten"=w135) -> ("Component Index out"=w130:i32, "Komponenten Index"=w133:u16)  [unwired: 7 in, 1 out]
        n57 = case shown="True" w139 {
          tunnel: w147 -> [w156 w177]
          tunnel: w146 -> [_ w176]
          tunnel: w145 -> [_ w175]
          tunnel: w144 -> [w155 w168]
          tunnel: [w152 w165] -> w143
          tunnel: [w151 w174] -> w142
          tunnel: [w156 w173] -> w141
          tunnel: w140 -> [_ w172]
          tunnel: w138 -> [_ w171]
          tunnel: w137 -> [w154 w167]
          tunnel: w136 -> [_ w169]
          tunnel: w133 -> [w153 w166]
          tunnel: w132 -> [_ w163]
          tunnel: w131 -> [_ w162]
          tunnel: w130 -> [w149 w159]
          tunnel: w129 -> [w150 w157]
          frame False {
            # "nur Stufentabelle\nspeichern"
            n58 = Bundle("SPAN Index"=w150, "Component Index out"=w149) -> (w148:T26)  [unwired: 1 in]
            n59 = call "set Stufentabelle.vi"("Index in"=w148, "Komponente in"=w153, "Table Index"=w154, "GD in"=w155) -> ("EGAK"=w151:T10[], "Stufen Tabellen out"=w152:string[][])  [unwired: 4 in, 2 out]
          }
          frame True {
            # "Ein- Ausgabe\nTabelle schreiben"
            n60 = Bundle("SPAN Index"=w157, "Component Index out"=w159) -> (w158:T26)  [unwired: 1 in]
            n61 = Equal?(x=w169, y=w167) -> (x = y?=w161:bool)
            n62 = Or(x=w161, y=w171) -> (x .or. y?=w170:bool)
            n63 = Bundle(w167, w158) -> (w160:T27)  [unwired: 1 in]
            n64 = Bundle(w170, w161, "Gesamtkonzentration"=w163, "höchste Konzentration Teilkomponente"=w162) -> (w164:T28)  [unwired: 1 in]
            n65 = call "Stufen abfragen Tabelle setzen und auslesen.vi"("E/A Cluster"=w164, "Ausgabetabelle (Eingang)"=w172, "GD Cluster"=w175, "Eingabetabelle (Eingang)"=w176, "Fehler (Eingang, kein Fehler)"=w177, "Komponente in"=w166, "Index Cluster"=w160, "GD in"=w168) -> ("Fehler (Ausgang)"=w173:errorcluster, "EGAK out"=w174:T10[], "Stufen Tabellen out"=w165:string[][])  [unwired: 1 out]
          }
        }
      }
      n66 = And(x=TRUE, y=w103) -> (x .and. y?=w101:bool)
      n67 = property class="Tbl (strikt)"(reference=w128, "Value"=w115) -> (error out=w126:errorcluster)  [unwired: 1 in, 1 out]
      n68 = property class="Arr (strikt)"(reference=w127, error in=w113, "Value"=w114) -> (error out=w125:errorcluster)  [unwired: 1 out]
      n69 = property class="Str (strikt)"(reference=w84, "Value"=w82) -> (error out=w85:errorcluster)  [unwired: 1 in, 1 out]
      n70 = case shown="True" w101 {
        tunnel: w107 -> [_ w196]
        tunnel: w106 -> [_ w195]
        frame False {
        }
        frame True {
          n71 = property class="Str"(reference=w196, "Value"=w195) -> (error out=w197:errorcluster)  [unwired: 1 in, 1 out]
          n72 = call <vilib>:"Clear Errors.vi"("error in (no error)"=w197) -> ()  [unwired: 5 in, 2 out]
        }
      }
      n73 = call <vilib>:"Clear Errors.vi"("error in (no error)"=w85) -> ()  [unwired: 5 in, 2 out]
      n74 = call <vilib>:"Clear Errors.vi"("error in (no error)"=w126) -> ()  [unwired: 5 in, 2 out]
      n75 = call <vilib>:"Clear Errors.vi"("error in (no error)"=w125) -> ("error out"=w112:errorcluster)  [unwired: 5 in, 1 out]
    }
  }
  n76 = Increment(x=w10) -> (x+1=w7:i32)
  n77 = call "Gasnummer in LIN Polynom setzen.vi"("Fehler (Eingang, kein Fehler)"=w9, "Gasnummer"=w7) -> ("Fehler (Ausgang)"=→"error out":errorcluster)  [unwired: 7 in, 2 out]
  "SpanInletClusterArray out" <- "SpanInletClusterArray in"
